vi "TestGaussianFit2D.vi"() -> ()   [LabVIEW 2009]
panel:
  in  "y0":dbl=35.0
  in  "x0":dbl=50.0
  in  "alpha":dbl[unit]=0.004886921905584123
  in  "b":dbl=0.2
  in  "a":dbl=0.1
  out "b":dbl format="%.2f"
  out "a":dbl format="%.2f"
  out "theta":dbl[unit] format="%.2f"
  out "y":dbl format="%.2f"
  out "x":dbl format="%.2f"
  out "Graphe d'intensité":dbl[][](graph)
  in  "Big Size":i32
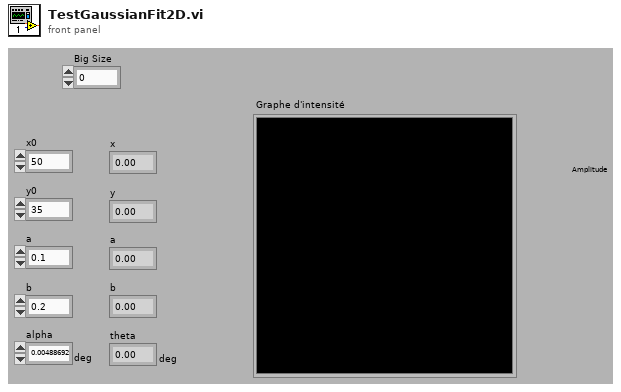
[diagram p1: front panel]
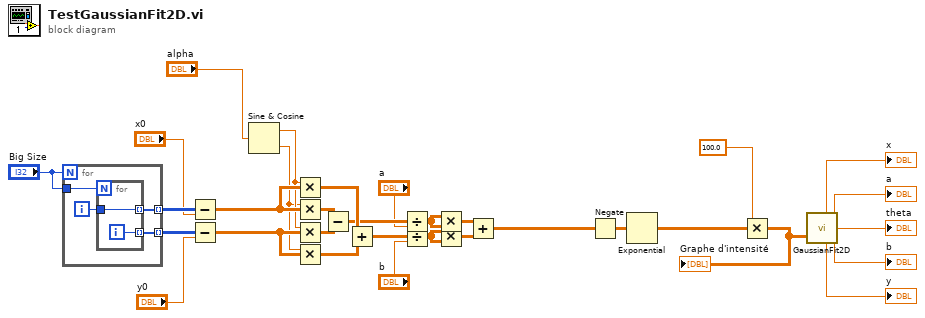
[diagram p0: block diagram]
diagram:
  n1 = for {
    N: "Big Size" -> [_]
    tunnel: "Big Size" -> [w36]
    tunnel: [w35] -> w30 mode=indexing
    tunnel: [w34] -> w31 mode=indexing
    i -> [w33]
    n2 = for {
      N: w36 -> [_]
      tunnel: [w38] -> w35 mode=indexing
      tunnel: [w37] -> w34 mode=indexing
      tunnel: w33 -> [w37]
      i -> [w38]
    }
  }
  n3 = Subtract(x=w31, y="x0") -> (x-y=w19:dbl[][])
  n4 = Subtract(x=w30, y="y0") -> (x-y=w18:dbl[][])
  n5 = Sine & Cosine(0:"alpha") -> (1:w17:dbl, 2:w16:dbl)
  n6 = Multiply(x=w17, y=w19) -> (x*y=w13:dbl[][])
  n7 = Multiply(x=w16, y=w19) -> (x*y=w15:dbl[][])
  n8 = Multiply(x=w17, y=w18) -> (x*y=w14:dbl[][])
  n9 = Multiply(x=w16, y=w18) -> (x*y=w12:dbl[][])
  n10 = Subtract(x=w15, y=w14) -> (x-y=w11:dbl[][])
  n11 = Add(x=w13, y=w12) -> (x+y=w10:dbl[][])
  n12 = Divide(x=w11, y="a") -> (x/y=w7:dbl[][])
  n13 = Divide(x=w10, y="b") -> (x/y=w6:dbl[][])
  n14 = Multiply(x=w7, y=w7) -> (x*y=w5:dbl[][])
  n15 = Multiply(x=w6, y=w6) -> (x*y=w4:dbl[][])
  n16 = Add(x=w5, y=w4) -> (x+y=w3:dbl[][])
  n17 = Negate(x=w3) -> (-x=w32:dbl[][])
  n18 = Exponential(1:w32) -> (0:w23:dbl[][])
  n19 = Multiply(x=100.0, y=w23) -> (x*y=w2:dbl[][])
  "Graphe d'intensité" <- w2
  n20 = call "GaussianFit2D.vi"("Image"=w2) -> ("b"=→"b":dbl, "y"=→"y":dbl, "theta"=→"theta":dbl[unit], "a"=→"a":dbl, "x"=→"x":dbl)  [unwired: 1 in]
